vi "Pseudo RT Doppler.vi"() -> ()   [LabVIEW 2022 SP3]
doc: "Acquire & Proc Scans - SW Trig is like the Acquire & Process N Scans example, but uses conditional retrieval to simulate analog triggering. It uses circular buffering and searches through the data as it is acquired until the trigger conditions have been met on the channel specified. The trigger channel must be one of the acquired channels. In this example retrieval (trigger) conditions can be changed as the example is running.\n\n\nBefore running this VI, set the values of the controls on the front panel. Select Show Help Window from the Help menu to see a description of each control. If the values you select for all the controls are values you will usually use, select Make Current Values Default from the Operate menu and save the VI. Or, you may save individual control's default values by popping up on the control, selecting Data Operations, then selecting Make Current Value Default, and saving the VI.\n\nThe buffer size is the number of scans that will be held in the internal memory buffer, and is limited by the amount of memory available. If you are acquiring a small, finite amount of data and can keep it all in memory, set buffer size to the number of scans to acquire. More often, you want to acquire more data than you can hold in memory, and you set the buffer size to hold a subset of the data, at least several seconds worth. Experiment with the buffer size and the number of scans to read each time. If the buffer is too small or you are not reading data from it fast enough, your data will be overwritten by new data before you have a chance to read it (overwrite error). If the buffer is too big, you will run out of memory (out of memory error).\n\nWhen you run this VI, it searches through acquired data in the buffer for the trigger conditions, then displays the data from all the channels on the graph as they are retrieved from the buffer, while the acquisition is still going on. Press the Stop button to stop the acquisition at any time."
uses:
  Doppler/dopplerV6.llb/AI Read (waveform).vi
panel:
  out "waveform graph":sgl[][](graph)
  in  "channels (0)":tag[](array[tag])=["I", "Q"]
  in  "input limits":cluster{"high limit":sgl, "low limit":sgl}[](array[cluster])=[{"high limit"=1.0, "low limit"=-1.0}] {"low limit" format="%.2f"; "high limit" format="%.2f"}
  out "timeout?":bool
  in  "interchannel delay\nin secs ( -1: hw default)":sgl=-1.0 format="%.2p"
  in  "hysteresis":sgl=0.01 format="%.2f"
  in  "time limit in sec\n(5 sec)":sgl=5.0 format="%.2f"
  in  "trigger level":sgl format="%.2f"
  in  "trig chan (0)":string="0"
  in  "pretrigger\nscans (0)":i32
  in  "trig slope (1:rising)":u16(ring)=1 items=["no change", "rising", "falling"]
  in  "scans to read\nat a time (1000)":i32=18000
  in  "scan rate\n(1000 scans/sec)":sgl=6000.0 format="%.2f"
  in  "device (1)":i16=1
  in  "stop":bool
  in  "buffer size\n(4000 scans)":i32=50000
  # "For instructions select File >> VI Properties >> Documentation"
  # "retrieval conditions"
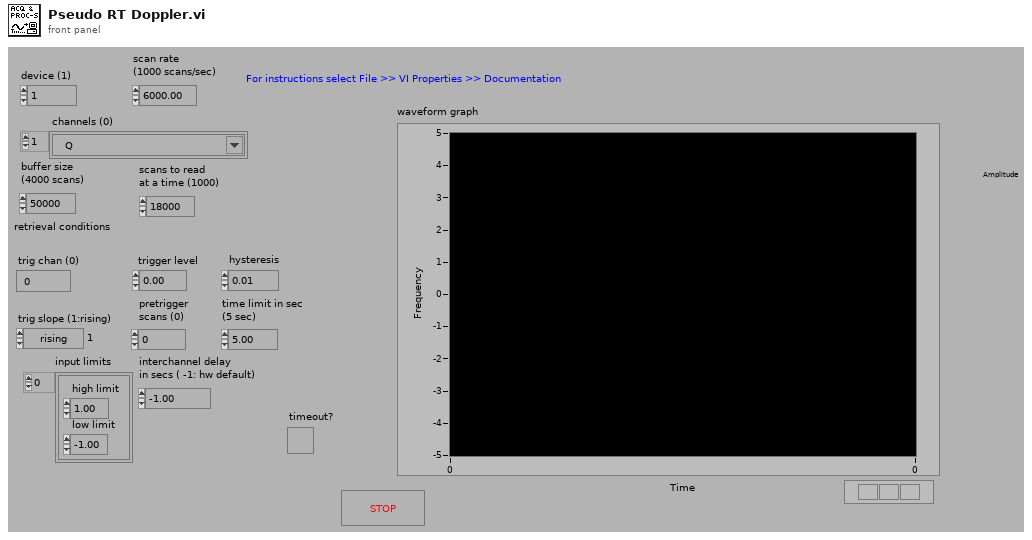
[diagram p1: front panel]
types:
  T1 = cluster{"read from end of data":i32, "read offset":i32}
  T2 = cluster{"conditional\nretrieval":i32, u32, "trig slope (1:rising)":u16, "trigger level":sgl, "hysteresis":sgl, u16, i32}
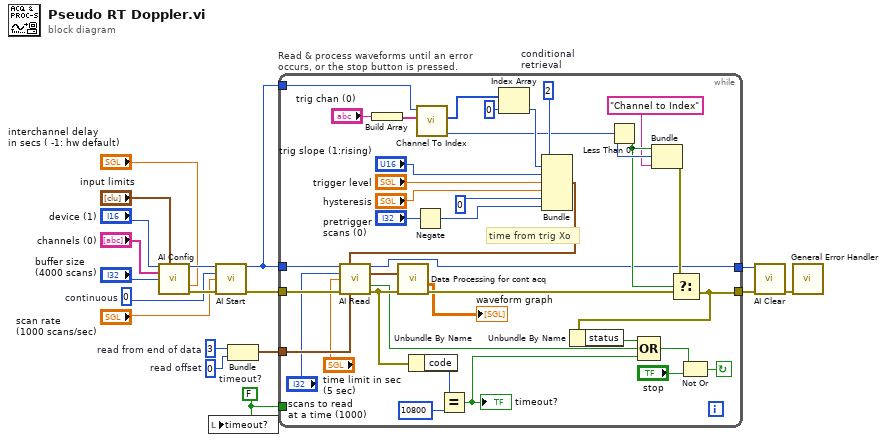
[diagram p0: block diagram]
diagram:
  w3 = FALSE  # timeout?
  w10 = 0  # read offset
  w11 = 3  # read from end of data
  w14 = 0  # continuous
  n1 = call "AI Config.vi"("device (1)"="device (1)", "input limits (no change)"="input limits", "channels (0)"="channels (0)", "buffer size (1000 scans)"="buffer size\n(4000 scans)", "interchannel delay (secs) (board default)"="interchannel delay\nin secs ( -1: hw default)") -> ("taskID"=w15:u32, "error out"=w18:errorcluster)  [unwired: 8 in, 1 out]
  n2 = local write "timeout?"(w3) -> ()
  n3 = call "AI Start.vi"("taskID in"=w15, "number of scans to acquire (-1)"=w14, "scan rate (1000 scans/sec)"="scan rate\n(1000 scans/sec)", "error in (no error)"=w18) -> ("taskID out"=w12:u32, "error out"=w17:errorcluster)  [unwired: 8 in, 2 out]
  n4 = Bundle("read from end of data"=w11, "read offset"=w10) -> (w9:T1)  [unwired: 1 in]
  n5 = while "Read & process waveforms until an error occurs, or the stop button is pressed." {
    tunnel: w12 -> [w46]
    tunnel: w17 -> [w55]
    tunnel: [w26] -> w5
    tunnel: [w20] -> w16
    tunnel: w12 -> [w45]
    tunnel: w9 -> [w43]
    tunnel: w3 -> [_]
    stop <- w54 continue-if-true
    w44 = 2  # conditional retrieval
    # "time from trig Xo"
    n6 = Build Array("trig chan (0)") -> (w48:string[])
    n7 = Negate(x="pretrigger\nscans (0)") -> (-x=w35:i32)
    n8 = call "Channel To Index.vi"("channel list"=w48, "task ID"=w45) -> ("status"=w30:i32, "channel indices"=w49:u32[])  [unwired: 7 in, 1 out]
    n9 = Index Array(array=w49, index=0) -> (element=w50:u32)
    n10 = Bundle("conditional\nretrieval"=w44, w50, "trig slope (1:rising)"="trig slope (1:rising)", "trigger level"="trigger level", "hysteresis"="hysteresis", u16 0, w35) -> (w47:T2)  [unwired: 1 in]
    n11 = call-poly "AI Read.vi"("taskID in"=w46, "conditional retrieval (off)"=w47, "number of scans to read (-1:all)"="scans to read\nat a time (1000)", "time limit in sec (-1:auto calculate)"="time limit in sec\n(5 sec)", "error in (no error)"=w55, "read/search position (from mark)"=w43) -> ("taskID out"=w20:u32, "waveform data"=w21:waveform(dbl)[], "retrieval complete"=w24:bool, "error out"=w33:errorcluster)  [unwired: 4 in, 2 out]
    n12 = call "Data Processing for cont acq.vi"("error in (no error)"=w33, "waveform"=w21) -> ("error out"=w31:errorcluster, "Intensity Graph"=→"waveform graph":sgl[][])  [unwired: 2 in, 2 out]
    n13 = Unbundle By Name(w33) -> ("code"=w32:i32)
    n14 = Equal?(x=w32, y=10800) -> (x = y?=w23:bool)
    "timeout?" <- w23
    n15 = Less Than 0?(x=w30) -> (x < 0?=w28:bool)
    n16 = Bundle(w28, "status"=w30, "Channel to Index") -> (w29:cluster{bool, "status":i32, string})  [unwired: 1 in]
    n17 = Select(t=w29, s=w28, f=w31) -> (s? t:f=w26:errorcluster)
    n18 = Unbundle By Name(w26) -> ("status"=w25:bool)
    n19 = Compound Arithmetic op=OR(w25, w24, w23) -> (w22:bool)
    n20 = Not Or(1:"stop", 2:w22) -> (0:w54:bool)
  }
  n21 = call "AI Clear.vi"("error in (no error)"=w5, "taskID in"=w16) -> ("error out"=w4:errorcluster)  [unwired: 4 in, 1 out]
  n22 = call <vilib>:"General Error Handler.vi"("error in (no error)"=w4) -> ()  [unwired: 10 in, 5 out]
